vi "NetComm_SendMessage.vi"(11 "Message":string) -> ()   [LabVIEW 2017]
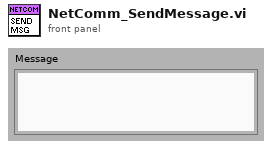
[diagram p1: front panel]
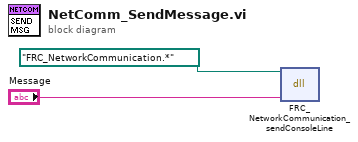
[diagram p0: block diagram]
diagram:
  n1 = dll-call lib="?" fn="FRC_NetworkCommunication_sendConsoleLine"(path in=path "FRC_NetworkCommunication.*", "message"="Message") -> ()  [unwired: 4 in, 2 out]
